vi "dfd_Create Multirate Filter.vi"(6 "fs":dbl=1.0, 8 "error in (no error)":errorcluster, 9 "mode":T2 items=["Default"=-1, "No Rate Change"=0, "Interpolation"=1, "Decimation"=2, "Interpolated"=3, "Rational"=4], 10 "factor":i32=1, 11 "h (n)":dbl[](array[numeric])) -> (0 "error out":errorcluster, 3 "multirate filter out":T1={"mMRate_Structure"=enum."CIC", "mMRate_Mode"=0, "mMRate_Factor"=1, "mMRate_FIRParams"={"mMRate_FIR_H"=[], "mMRate_FIR_IsNyquist?"=FALSE, "mMRate_FIR_IsSymmetric?"=FALSE}, "mMRate_CICParams"={"mMRate_CIC_#Stage"=2, "mMRate_CIC_Lag"=1, "mMRate_CIC_Type"=enum."Lowpass"}, "mMRate_Order"=1, "mMRate_Version"="1.0", "mMRate_Comments"="1.0", "mMRate_RationalFactor"={"mMRate_L"=-1, "mMRate_M"=-1}, "mMRate_Fs"=1.0, "mMRate_Quantized?"=FALSE, "mMRate_QFilterGain"=1.0, "mMRate_CoefWl"=16, "mMRate_Scaling"={"mMRate_ScaleByPowerOf2?"=FALSE, "mMRate_ScaleType"=enum."Time Domain 1-Norm"}, "mMRate_InputWl"=0, "mMRate_OutputWl"=0, "mMRate_OutputMode"=enum."Nearest", "mMRate_MultMode"=enum."Full", "mMRate_BitPruning"=FALSE, "mMRate_GainWl"=16, "mMRate_OutputFwl"=0, "mMRate_SumIwl"=0, "mMRate_InputIwl "=16, "mMRate_SumWl"=32, "mMRate_CoefIwl"=0} {"mMRate_SumWl" min=1 max=32 step=1; "mMRate_InputIwl" min=1 max=32 step=1; "mMRate_GainWl" min=1 max=32 step=1; "mMRate_OutputWl" min=1 max=32 step=1; "mMRate_InputWl" min=1 max=32 step=1; "mMRate_CoefWl" min=1 max=32 step=1; "mMRate_Mode" items=["Default"=-1, "No Rate Change"=0, "Interpolation"=1, "Decimation"=2, "Interpolated"=3, "Rational"=4]})   [LabVIEW 2017, in "NI_DigFilterLicensed.lvlib"]
uses:
  <vilib>/addons/Digital Filter Design/NI_DigFilterLicensed.lvlib
  <vilib>/addons/Digital Filter Design/_Objects.llb/DFD Multirate Mode.ctl
  <vilib>/addons/Digital Filter Design/_Objects.llb/DFD Multirate Filter Obj.ctl
  <vilib>/addons/Digital Filter Design/_Objects.llb/DFD Coef Norm Type.ctl
  <vilib>/addons/Digital Filter Design/_Objects.llb/DFD Round-off Mode.ctl
  <vilib>/addons/Digital Filter Design/_Objects.llb/DFD FXP MRate Multiply Mode.ctl
  <vilib>/addons/Digital Filter Design/_Misc.llb/dfd_Error Handlers (Multiple).vi
panel:
  in  "multirate filter":T1={"mMRate_Structure"=enum."IIR", "mMRate_Mode"=0, "mMRate_Factor"=-1, "mMRate_FIRParams"={"mMRate_FIR_H"=[], "mMRate_FIR_IsNyquist?"=FALSE, "mMRate_FIR_IsSymmetric?"=FALSE}, "mMRate_CICParams"={"mMRate_CIC_#Stage"=0, "mMRate_CIC_Lag"=0, "mMRate_CIC_Type"=enum."Lowpass"}, "mMRate_Order"=0, "mMRate_Version"="2.0", "mMRate_Comments"="", "mMRate_RationalFactor"={"mMRate_L"=-1, "mMRate_M"=-1}, "mMRate_Fs"=1.0, "mMRate_Quantized?"=FALSE, "mMRate_QFilterGain"=1.0, "mMRate_CoefWl"=16, "mMRate_Scaling"={"mMRate_ScaleByPowerOf2?"=FALSE, "mMRate_ScaleType"=enum."No Norm"}, "mMRate_InputWl"=16, "mMRate_OutputWl"=16, "mMRate_OutputMode"=enum."Truncation", "mMRate_MultMode"=enum."Truncated", "mMRate_BitPruning"=FALSE, "mMRate_GainWl"=16, "mMRate_OutputFwl"=0, "mMRate_SumIwl"=0, "mMRate_InputIwl "=16, "mMRate_SumWl"=32, "mMRate_CoefIwl"=0} {"mMRate_SumWl" min=1 max=32 step=1; "mMRate_InputIwl" min=1 max=32 step=1; "mMRate_GainWl" min=1 max=32 step=1; "mMRate_OutputWl" min=1 max=32 step=1; "mMRate_InputWl" min=1 max=32 step=1; "mMRate_CoefWl" min=1 max=32 step=1; "mMRate_Mode" items=["Default"=-1, "No Rate Change"=0, "Interpolation"=1, "Decimation"=2, "Interpolated"=3, "Rational"=4]}
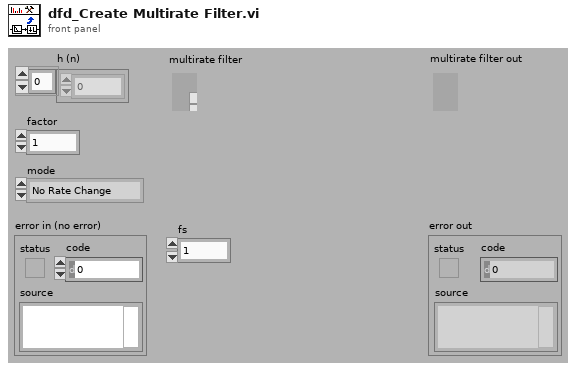
[diagram p1: front panel]
types:
  T1 = typedef "NI_DigFilterLicensed.lvlib/DFD Multirate Filter Obj.ctl" = cluster{"mMRate_Structure":enum16{"CIC", "FIR", "IIR", "Lattice"}, "mMRate_Mode":T2, "mMRate_Factor":i32, "mMRate_FIRParams":cluster{"mMRate_FIR_H":dbl[], "mMRate_FIR_IsNyquist?":bool, "mMRate_FIR_IsSymmetric?":bool}, "mMRate_CICParams":cluster{"mMRate_CIC_#Stage":i32, "mMRate_CIC_Lag":i32, "mMRate_CIC_Type":enum16{"Lowpass", "Highpass"}}, "mMRate_Order":i32, "mMRate_Version":string, "mMRate_Comments":string, "mMRate_RationalFactor":cluster{"mMRate_L":i32, "mMRate_M":i32}, "mMRate_Fs":dbl, "mMRate_Quantized?":bool, "mMRate_QFilterGain":dbl, "mMRate_CoefWl":i16, "mMRate_Scaling":cluster{"mMRate_ScaleByPowerOf2?":bool, "mMRate_ScaleType":T3}, "mMRate_InputWl":i16, "mMRate_OutputWl":i16, "mMRate_OutputMode":T4, "mMRate_MultMode":T5, "mMRate_BitPruning":bool, "mMRate_GainWl":i16, "mMRate_OutputFwl":i16, "mMRate_SumIwl":i16, "mMRate_InputIwl ":i16, "mMRate_SumWl":i16, "mMRate_CoefIwl":i16}
  T2 = typedef "NI_DigFilterLicensed.lvlib/DFD Multirate Mode.ctl" = i16
  T3 = typedef "NI_DigFilterLicensed.lvlib/DFD Coef Norm Type.ctl" = enum16{"No Norm", "Time Domain 1-Norm", "Time Domain 2-Norm", "Time Domain Inf-Norm"}
  T4 = typedef "NI_DigFilterLicensed.lvlib/DFD Round-off Mode.ctl" = enum16{"Nearest", "Truncation"}
  T5 = typedef "NI_DigFilterLicensed.lvlib/DFD FXP MRate Multiply Mode.ctl" = enum16{"Truncated", "Full"}
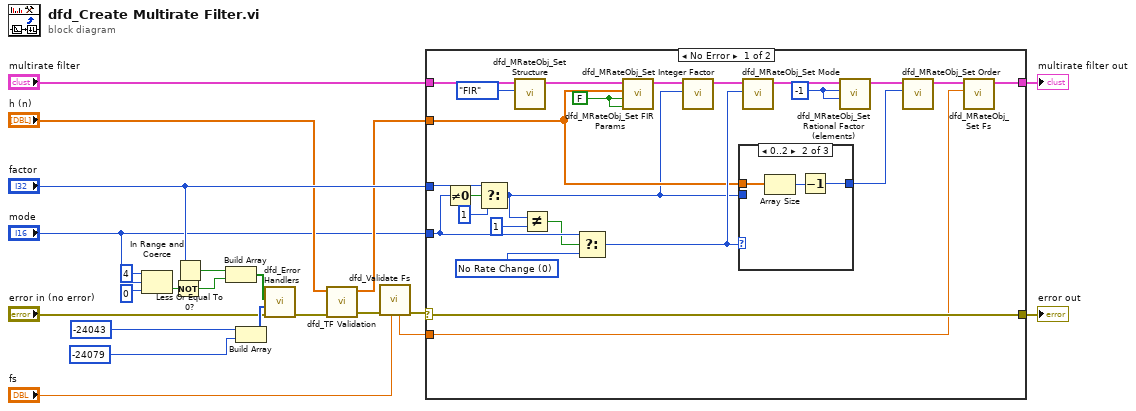
[diagram p0: block diagram]
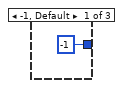
[diagram p2: hidden frame]
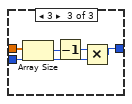
[diagram p3: hidden frame]
diagram:
  n1 = In Range and Coerce(upper limit=i16 4, x="mode", lower limit=i16 0) -> (In Range?=w13:bool)  [unwired: 1 out]
  n2 = Not(x=w13) -> (.not. x?=w11:bool)
  n3 = Less Or Equal To 0?(x="factor") -> (x <= 0?=w16:bool)
  n4 = Build Array(w16, w11) -> (w12:bool[])
  n5 = Build Array(-24043 ("ERR_FACTOR_LE_ZERO"), -24079 ("ERR_FILTERING_MODE")) -> (w10:i32[])
  n6 = call-poly <vilib>:"dfd_Error Handlers.vi"("error in (no error)"="error in (no error)", "error sources"=w10, "condition failed?"=w12) -> ("error out"=w15:errorcluster)  [unwired: 8 out]
  n7 = call <vilib>:"dfd_TF Validation.vi"("error in (no error)"=w15, "numerator"="h (n)") -> ("error out"=w5:errorcluster, "validated numerator"=w17:dbl[])  [unwired: 1 in, 4 out]
  n8 = call <vilib>:"dfd_Validate Fs.vi"("fs [Hz]"="fs", "error in (no error)"=w5) -> ("error out"=w4:errorcluster, "dup fs [Hz]"=w1:dbl)  [unwired: 8 in]
  n9 = case shown="No Error" w4 {
    selector: w4 -> [w46 w57]
    tunnel: "mode" -> [w42 _]
    tunnel: "factor" -> [w43 _]
    tunnel: w17 -> [w30 _]
    tunnel: "multirate filter" -> [w37 w56]
    tunnel: [w41 w56] -> w19
    tunnel: [w46 w57] -> w20
    tunnel: w1 -> [w23 _]
    frame No Error {
      w40 = T2 0 items=["Default"=-1, "No Rate Change"=0, "Interpolation"=1, "Decimation"=2, "Interpolated"=3, "Rational"=4] ("f")
      w38 = FALSE ("is Nyquist?")
      w33 = -1 ("rational factor.L")
      n10 = Not Equal To 0?(x=w42) -> (x != 0?=w45:bool)
      n11 = Select(t=w43, s=w45, f=1) -> (s? t:f=w27:i32)
      n12 = call <vilib>:"dfd_MRateObj_Set Structure.vi"("structure"=enum16{"CIC", "FIR", "IIR", "Lattice"}."FIR", "multirate filter in"=w37) -> ("multirate filter out"=w25:T1)  [unwired: 9 out]
      n13 = Not Equal?(x=w27, y=1 ("x")) -> (x != y?=w28:bool)
      n14 = Select(t=w42, s=w28, f=w40) -> (s? t:f=w35:T2)
      n15 = call <vilib>:"dfd_MRateObj_Set FIR Params.vi"("is symmetric?"=w38, "is Nyquist?"=w38, "h(n)"=w30, "multirate filter in"=w25) -> ("multirate filter out"=w24:T1)  [unwired: 7 out]
      n16 = call <vilib>:"dfd_MRateObj_Set Integer Factor.vi"("factor"=w27, "multirate filter in"=w24) -> ("multirate filter out"=w36:T1)  [unwired: 9 out]
      n17 = case shown="0..2" w35 {
        tunnel: w30 -> [_ w50 w55]
        tunnel: w27 -> [_ _ w52]
        tunnel: [-1 w48 w51] -> w26
        frame -1, Default {
        }
        frame 0..2 {
          n18 = Array Size(array=w50) -> (size(s)=w49:i32)
          n19 = Decrement(x=w49) -> (x-1=w48:i32)
        }
        frame 3 {
          n20 = Array Size(array=w55) -> (size(s)=w54:i32)
          n21 = Decrement(x=w54) -> (x-1=w53:i32)
          n22 = Multiply(x=w53, y=w52) -> (x*y=w51:i32)
        }
      }
      n23 = call <vilib>:"dfd_MRateObj_Set Mode.vi"("mode"=w35, "multirate filter in"=w36) -> ("multirate filter out"=w34:T1)  [unwired: 9 out]
      n24 = call <vilib>:"dfd_MRateObj_Set Rational Factor (elements).vi"("M"=w33, "L"=w33, "multirate filter in"=w34) -> ("multirate filter out"=w32:T1)  [unwired: 8 out]
      n25 = call <vilib>:"dfd_MRateObj_Set Order.vi"("order"=w26, "multirate filter in"=w32) -> ("multirate filter out"=w31:T1)  [unwired: 9 out]
      n26 = call <vilib>:"dfd_MRateObj_Set Fs.vi"("fs"=w23, "multirate filter in"=w31) -> ("dup multirate filter"=w41:T1)  [unwired: 9 out]
    }
    frame Error {
    }
  }
  "error out" <- w20
  "multirate filter out" <- w19
